vi "Get Stimulus Fit.vi"(8 "error in (no error)":errorcluster, 11 "Halfwave Sinusoidal Fit in":refnum<class "Halfwave Sinusoidal Fit.lvclass">) -> (0 "error out":errorcluster, 2 "Fit out":dbl[](array[numeric]), 3 "Halfwave Sinusoidal Fit out":refnum<class "Halfwave Sinusoidal Fit.lvclass">)   [LabVIEW 2016, in "Halfwave Sinusoidal Fit.lvclass"]
uses:
  Halfwave Sinusoidal Fit.lvclass
  Sinusoidal Fit.lvclass
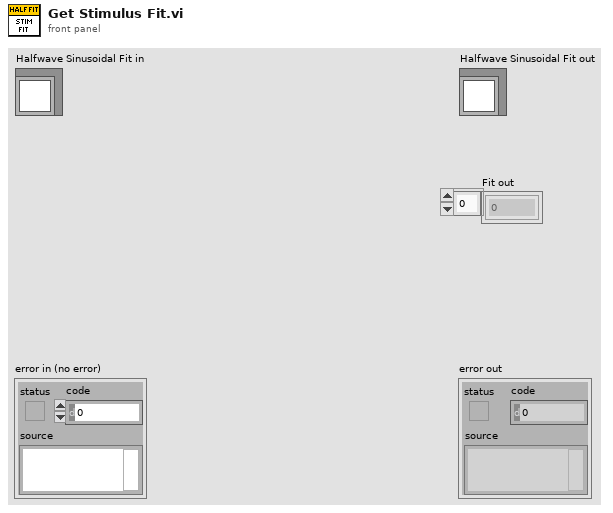
[diagram p1: front panel]
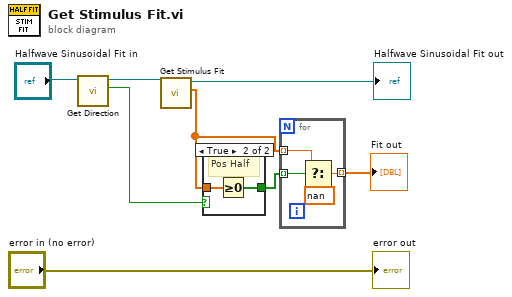
[diagram p0: block diagram]
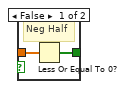
[diagram p2: hidden frame]
diagram:
  n1 = call-dynamic "Get Direction.vi"("Halfwave Sinusoidal Fit in"="Halfwave Sinusoidal Fit in") -> ("Direction"=w4:bool, "Halfwave Sinusoidal Fit out"=w5:refnum<class "Halfwave Sinusoidal Fit.lvclass">)  [unwired: 8 in, 1 out]
  n2 = call-parent "Get Stimulus Fit.vi"("Sinusoidal Fit in"=w5) -> ("Fit out"=w3:dbl[], "Sinusoidal Fit out"=→"Halfwave Sinusoidal Fit out":refnum<class "Halfwave Sinusoidal Fit.lvclass">)  [unwired: 8 in, 1 out]
  n3 = case shown="True" w4 {
    tunnel: w3 -> [w9 w12]
    tunnel: [w10 w11] -> w2
    frame False {
      # "Neg Half"
      n4 = Less Or Equal To 0?(x=w9) -> (x <= 0?=w10:bool[])
    }
    frame True {
      # "Pos Half"
      n5 = Greater Or Equal To 0?(x=w12) -> (x >= 0?=w11:bool[])
    }
  }
  n6 = for {
    tunnel: w2 -> [w13] mode=indexing
    tunnel: w3 -> [w16] mode=indexing
    tunnel: [w14] -> w1 mode=indexing
    n7 = Select(t=w16, s=w13, f=nan) -> (s? t:f=w14:dbl)
  }
  "Fit out" <- w1
  "error out" <- "error in (no error)"
